vi "Read VIs Module Interface from Front Panel.vi"(8 "error in":errorcluster, 11 "VI in":refnum<vi>) -> (0 "error out":errorcluster, 3 "Map":map{string, variant}(c390))   [LabVIEW 2025]
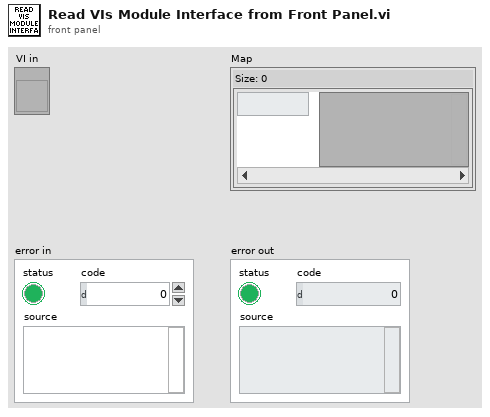
[diagram p1: front panel]
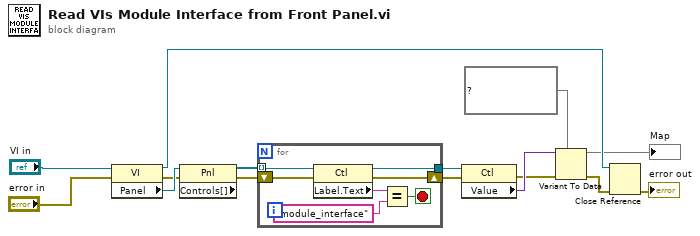
[diagram p0: block diagram]
diagram:
  n1 = property class="VI"(reference="VI in", error in="error in") -> (reference out=w15:refnum<vi>, error out=w6:errorcluster, "Panel"=w8:refnum<vi>)
  n2 = property class="Pnl"(reference=w8, error in=w6) -> (error out=w3:errorcluster, "Controls[]"=w7:refnum<vi>[])  [unwired: 1 out]
  n3 = for {
    tunnel: w7 -> [w22] mode=indexing
    tunnel: [w19] -> w9
    shift-right: [w17] -> w4
    shift-left: w3 -> [w16]
    stop <- w18 stop-if-true
    n4 = property class="Ctl"(reference=w22, error in=w16) -> (reference out=w19:refnum<vi>, error out=w17:errorcluster, "Label.Text"=w21:string)
    n5 = Equal?(x=w21, y="module_interface") -> (x = y?=w18:bool)
  }
  n6 = property class="Ctl"(reference=w9, error in=w4) -> (error out=w5:errorcluster, "Value"=w10:variant)  [unwired: 1 out]
  n7 = Variant To Data(error in=w5, type=map{string, variant} {} ("Size: 0"), Variant=w10) -> (data=→"Map":map{string, variant}, error out=w2:errorcluster)
  n8 = Close Reference(reference=w15, error in (no error)=w2) -> (error out=→"error out":errorcluster)
